vi "Is Data Ready.vi"(8 "error in (no error)":errorcluster, 11 "Ni-Scope Digitizer in":refnum<class "Ni-Scope Digitizer.lvclass">) -> (0 "error out":errorcluster, 1 "Data ready":bool, 2 "Availiable Samples":u32, 3 "Ni-Scope Digitizer out":refnum<class "Ni-Scope Digitizer.lvclass">)   [LabVIEW 2016, in "Ni-Scope Digitizer.lvclass"]
uses:
  Ni-Scope Digitizer.lvclass
  C:/github/NHMFL_Core/Libraries/Instruments/Pulse Driver/Pulse Driver.lvclass
  Ni-Scope Digitizer.lvclass/Ni-Scope Digitizer.ctl
  Instruments/Pulse Driver/Pulse Driver.lvclass/Pulse Driver.ctl
  Read instrument handle.vi
  Instruments/Pulse Driver/Read Samples per read.vi
  Instruments/Pulse Driver/Read Samples per channel.vi
  Write instrument handle.vi
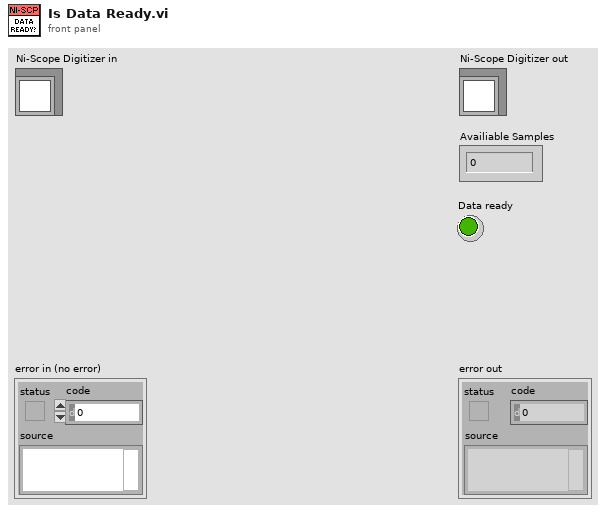
[diagram p1: front panel]
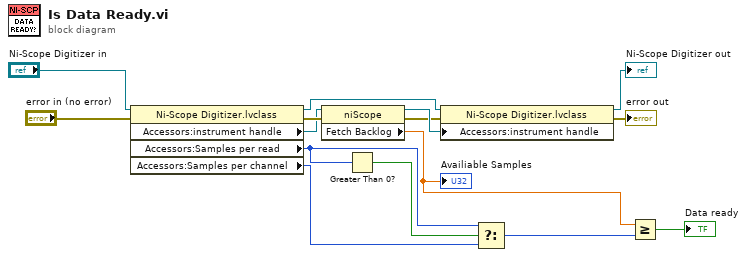
[diagram p0: block diagram]
diagram:
  n1 = property class="Ni-Scope Digitizer.lvclass"(reference="Ni-Scope Digitizer in", error in="error in (no error)") -> (reference out=w5:refnum<class "Ni-Scope Digitizer.lvclass">, error out=w8:errorcluster, "Accessors:instrument handle"=w6:refnum<k15>, "Accessors:Samples per read"=w7:i32, "Accessors:Samples per channel"=w11:i32)
  n2 = property class="niScope"(reference=w6, error in=w8) -> (reference out=w3:refnum<k15>, error out=w2:errorcluster, "Fetch Backlog"=w15:dbl)
  "Availiable Samples" <- w15
  n3 = Greater Than 0?(x=w7) -> (x > 0?=w12:bool)
  n4 = property class="Ni-Scope Digitizer.lvclass"(reference=w5, error in=w2, "Accessors:instrument handle"=w3) -> (reference out=→"Ni-Scope Digitizer out":refnum<class "Ni-Scope Digitizer.lvclass">, error out=→"error out":errorcluster)
  n5 = Select(t=w7, s=w12, f=w11) -> (s? t:f=w10:i32)
  n6 = Greater Or Equal?(x=w15, y=w10) -> (x >= y?=→"Data ready":bool)
